vi "macro_vecBuilder_ArrayBy1FIll.vi"   [LabVIEW 2019, in "Trajectory_Library.lvlib"]
uses:
  Trajectory_Library.lvlib
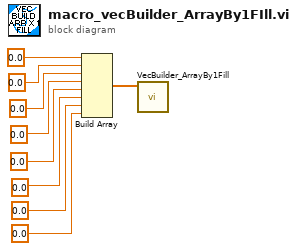
[diagram p0: block diagram]
diagram:
  n1 = Build Array(0.0 ("R0"), 0.0 ("R1"), 0.0 ("R2"), 0.0 ("R3"), 0.0 ("R4"), 0.0 ("R5"), 0.0 ("R6"), 0.0 ("R7")) -> (w9:dbl[])
  n2 = call "VecBuilder_ArrayBy1Fill.vi"("R Array"=w9) -> ()  [unwired: 10 in, 1 out]
